vi "SPI_Init_Device.vi"(1 "ClockDivisor":u32 max=65535 step=1, 2 "Handle":u32) -> (0 "FTC_Status":u32)   [LabVIEW 2010]
uses:
  WINNT/system32/FTCSPI.dll
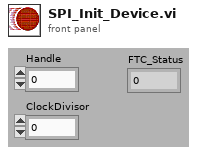
[diagram p1: front panel]
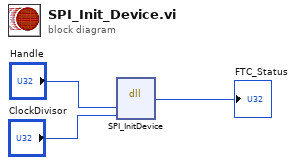
[diagram p0: block diagram]
diagram:
  n1 = dll-call lib="C:/Users/WINNT/system32/FTCSPI.dll" fn="SPI_InitDevice"("Handle"="Handle", "ClockDivisor"="ClockDivisor") -> ("FTC_Status"=→"FTC_Status":u32)  [unwired: 5 in, 2 out]
